vi "getMEDFilterStatus.vi.vi"(8 "error in (no error)":errorcluster, 10 "Measurement Function (0: Current)":T2 items=["Current", "Charge", "Voltage", "Resistance"], 11 "Electrometer in":refnum<class "Electrometer.lvclass">) -> (0 "error out":errorcluster, 1 "readOK?":bool, 2 "Filter type":T1, 3 "Electrometer out":refnum<class "Electrometer.lvclass">)   [LabVIEW 2016, in "Electrometer.lvclass"]
uses:
  Electrometer.lvclass
  Modes.ctl
  MED Filter Type.ctl
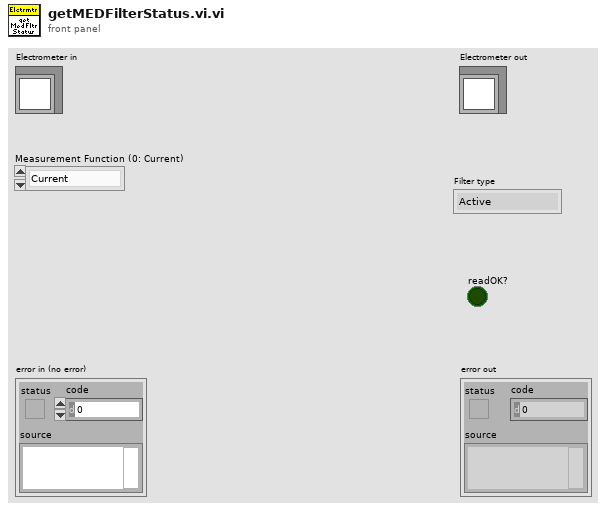
[diagram p1: front panel]
types:
  T1 = typedef "Electrometer.lvclass/MED Filter Type.ctl" = enum16{"Active", "None"}
  T2 = typedef "Electrometer.lvclass/Modes.ctl" = i32
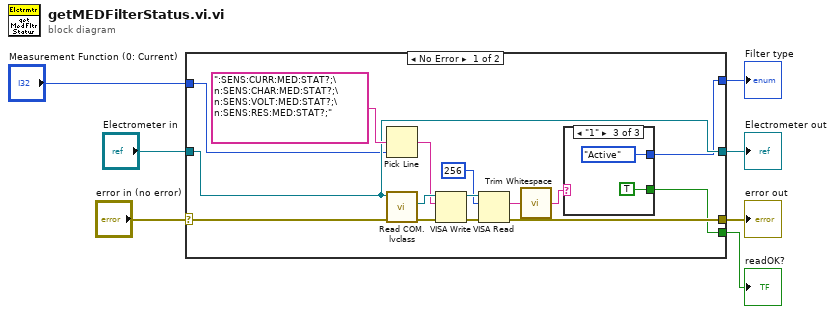
[diagram p0: block diagram]
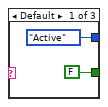
[diagram p2: hidden frame]
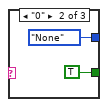
[diagram p3: hidden frame]
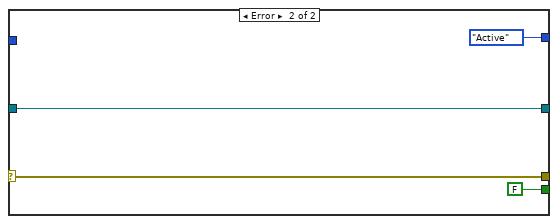
[diagram p4: hidden frame]
diagram:
  n1 = case shown="No Error" "error in (no error)" {
    selector: "error in (no error)" -> [w18 w32]
    tunnel: [w14 w32] -> w6
    tunnel: [w17 w31] -> w4
    tunnel: "Electrometer in" -> [w17 w31]
    tunnel: "Measurement Function (0: Current)" -> [w16 _]
    tunnel: [w11 MED_Filter_Type."Active" ("Filter")] -> w2
    tunnel: [w10 FALSE ("readOK?")] -> w1
    frame No Error {
      n2 = Pick Line(multi-line string=":SENS:CURR:MED:STAT?;\n:SENS:CHAR:MED:STAT?;\n:SENS:VOLT:MED:STAT?;\n:SENS:RES:MED:STAT?;", line index=w16) -> (output string=w19:string)  [unwired: 1 in]
      n3 = call "Read COM.lvclass.vi"("error in (no error)"=w18, "Electrometer in"=w17) -> ("error out"=w20:errorcluster, "VISA"=w22:refnum<visa-resource-name>)  [unwired: 7 in, 1 out]
      n4 = VISA Write(VISA resource name=w22, write buffer=w19, error in (no error)=w20) -> (VISA resource name out=w13:refnum<visa-resource-name>, error out=w15:errorcluster)  [unwired: 1 out]
      n5 = VISA Read(VISA resource name=w13, byte count=u32 256, error in (no error)=w15) -> (read buffer=w8:string, error out=w14:errorcluster)  [unwired: 2 out]
      n6 = call <vilib>:"Trim Whitespace.vi"("string"=w8) -> ("trimmed string"=w9:string)  [unwired: 1 in]
      n7 = case shown="\"1\"" w9 {
        tunnel: [MED_Filter_Type."Active" ("Filter") MED_Filter_Type."None" ("Filter") MED_Filter_Type."Active" ("Filter")] -> w11
        tunnel: [FALSE ("readOK?") TRUE ("readOK?") TRUE ("readOK?")] -> w10
        frame Default {
        }
        frame "0" {
        }
        frame "1" {
        }
      }
    }
    frame Error {
    }
  }
  "error out" <- w6
  "Electrometer out" <- w4
  "Filter type" <- w2
  "readOK?" <- w1
